vi "Write_UV_Lamp.vi"(0 "Refnum in":refnum<k21>, 1 "On/Off":bool, 5 "error in (no error)":errorcluster) -> (14 "Refnum out":refnum<k21>, 19 "error out":errorcluster)   [LabVIEW 2013]
uses:
  <vilib>/DAQmx/write.llb/DAQmx Write (Digital Bool 1Line 1Point).vi
  <vilib>/DAQmx/miscellaneous.llb/DAQmx Fill In Error Info.vi
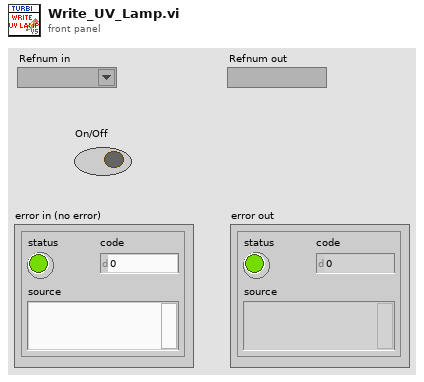
[diagram p1: front panel]
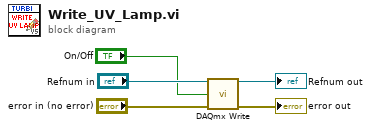
[diagram p0: block diagram]
diagram:
  n1 = call-poly <vilib>:"DAQmx Write.vi"("task/channels in"="Refnum in", "data"="On/Off", "error in"="error in (no error)") -> ("task out"=→"Refnum out":refnum<k21>, "error out"=→"error out":errorcluster)  [unwired: 10 in, 1 out]
